vi "Tracking.vi"(4 "Offset Home 2 RCM":dbl[](array[numeric])=[0.0, 0.0, 0.0, 0.0], 5 "Trajectory Cluster":T3, 6 "PID Cluster":T6={"L1 to L4 PID Cluster"={"L1 PID Gains"={"Kp"=0.005, "Kd"=0.5, "Ki"=0.0005}, "L2 PID Gains"={"Kp"=0.01, "Kd"=1.0, "Ki"=0.005}, "L3 PID Gains"={"Kp"=0.05, "Kd"=1.0, "Ki"=0.0005}, "L4 PID Gains"={"Kp"=0.1, "Kd"=0.1, "Ki"=0.0005}}, "Stage PID Cluster"={"Stage Z PID"={"Kp"=0.0005, "Kd"=0.001, "Ki"=0.0}, "Stage Y PID"={"Kp"=0.0003, "Kd"=0.01, "Ki"=0.0}, "Stage X PID"={"Kp"=0.0003, "Kd"=0.01, "Ki"=0.0}}, "OCT Z PID Gains"={"Kp"=0.0003, "Kd"=0.0001, "Ki"=0.01}}, 7 "Eye Model Cluster":T2={"X Grid"=[], "Y Grid"=[], "Za_true Surf"=[], "Iris Center"=[], "Zp_true Surf"=[], "Pinv"=[[1.0, 0.0], [0.0, 1.0]], "za_true"=5.0, "za_work"=1.0, "zp_work"=-1.0, "zp_true"=-5.0}, 8 "error in":errorcluster, 9 "Resume Index":i32, 10 "Prev Posit Cluster":T5={"Prev L1 to L4 Posit"=[-0.5319, -0.035669172703475985, -2.0566170657346783, 0.9099264705882353], "Prev Stage Posit"=[6.002553885707208, 5.996566124542428, 5.995469940427586], "Prev OCT Z Posit"=-0.0}, 11 "FPGA VI Reference In":refnum<k20>) -> (0 "error out":errorcluster, 1 "Leave Index":i32, 2 "Last Posit Cluster":T4={"Last L1 to L4 Posit"=[0.0, 0.0, 0.0, 0.0], "Last Stage Posit"=[6.0, 6.0, 6.0], "Last OCT Z Posit"=0.0}, 3 "FPGA VI Reference Out":refnum<k20>)   [LabVIEW 2016]
uses:
  <vilib>/Analysis/Matrix/Datatypes/RealMatrix.ctl
  <vilib>/Platform/TimedLoop/XDataNode/timing_clust.ctl
  <vilib>/Platform/TimedLoop/XDataNode/nitl_modes.ctl
  <vilib>/Platform/TimedLoop/XDataNode/wakeup.ctl
  Global Variables.vi
  <vilib>/platform/TimedLoop/XDataNode/XDataNode.xnode
  <vilib>/Platform/TimedLoop/XDataNode/XDNodeRunTimeDep.lvlib
  Library/KevinLibraryAll/labview/KevLib01.lvlib
  <vilib>/Analysis/Matrix/NI_Matrix.lvlib
panel:
  out "PC z Displacement":dbl
  out "Speed Schedule":dbl
  out "In Servo Loop":bool
  out "joint limits":dbl[][](array[numeric])=[[-10.0, 35.0], [-35.0, 35.0], [0.1, 10.0], [-40.0, 40.0]]
  out "Vac Extremum":dbl[](array[numeric])
  out "z Dist Thld":dbl[](array[numeric])
  out "z Rot Axis":dbl
  out "Deform Array":dbl[](array[numeric])=[1.0, 1.0, 1.0, 0.0, 0.0, 0.0, 0.0, 0.0, 0.0]
  out "Speed Override":u16(ring)=3 items=["4x", "3x", "2x", "1x", "0.5x", "0.2x", "0.1x", "PAUSE"]
  out "Loading Finished":bool
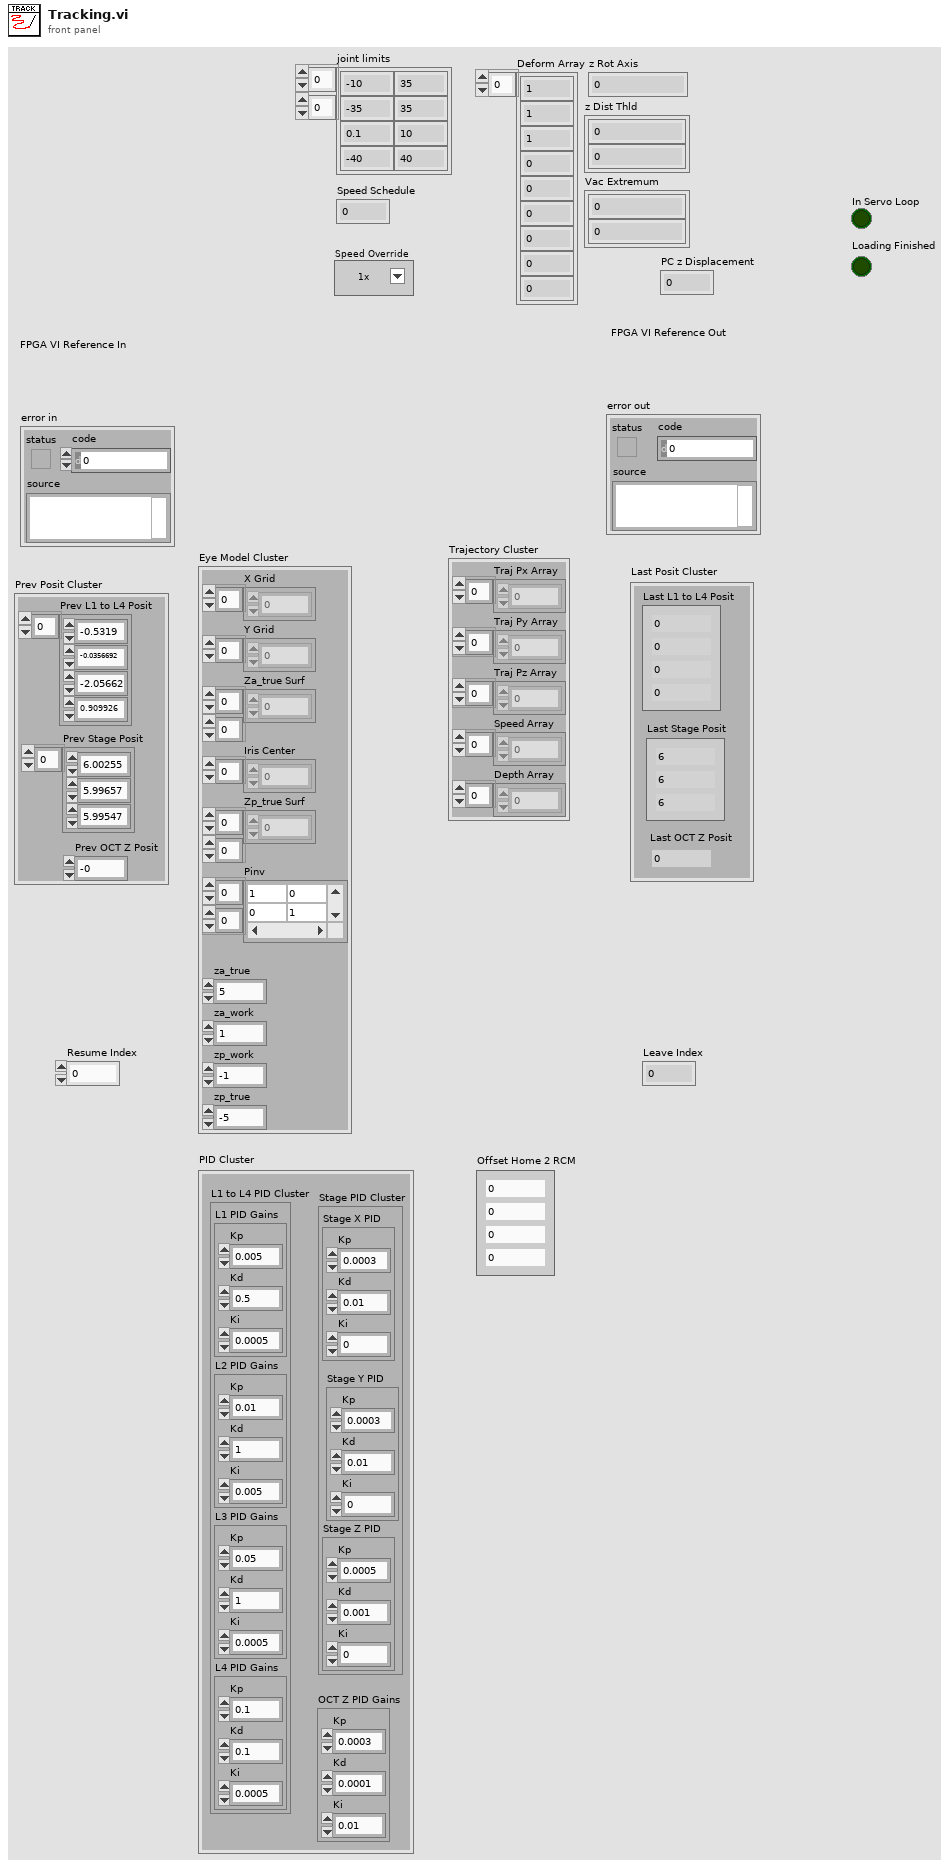
[diagram p1: front panel]
types:
  T1 = typedef "NI_Matrix.lvlib/RealMatrix.ctl" = dbl[][]
  T2 = cluster{"X Grid":dbl[], "Y Grid":dbl[], "Za_true Surf":dbl[][], "Iris Center":dbl[], "Zp_true Surf":dbl[][], "Pinv":T1, "za_true":dbl, "za_work":dbl, "zp_work":dbl, "zp_true":dbl}
  T3 = cluster{"Traj Px Array":dbl[], "Traj Py Array":dbl[], "Traj Pz Array":dbl[], "Speed Array":dbl[], "Depth Array":dbl[]}
  T4 = cluster{"Last L1 to L4 Posit":dbl[], "Last Stage Posit":dbl[], "Last OCT Z Posit":dbl}
  T5 = cluster{"Prev L1 to L4 Posit":dbl[], "Prev Stage Posit":dbl[], "Prev OCT Z Posit":dbl}
  T6 = cluster{"L1 to L4 PID Cluster":cluster{"L1 PID Gains":cluster{"Kp":dbl, "Kd":dbl, "Ki":dbl}, "L2 PID Gains":cluster{"Kp":dbl, "Kd":dbl, "Ki":dbl}, "L3 PID Gains":cluster{"Kp":dbl, "Kd":dbl, "Ki":dbl}, "L4 PID Gains":cluster{"Kp":dbl, "Kd":dbl, "Ki":dbl}}, "Stage PID Cluster":cluster{"Stage Z PID":cluster{"Kp":dbl, "Kd":dbl, "Ki":dbl}, "Stage Y PID":cluster{"Kp":dbl, "Kd":dbl, "Ki":dbl}, "Stage X PID":cluster{"Kp":dbl, "Kd":dbl, "Ki":dbl}}, "OCT Z PID Gains":cluster{"Kp":dbl, "Kd":dbl, "Ki":dbl}}
  T7 = typedef "XDNodeRunTimeDep.lvlib/timing_clust.ctl" = cluster{"Expected End [f-1]":u64, "Actual End [f-1]":u64, "Finished Late? [f-1]":bool, "Expected End [i-1]":u64, "Actual End [i-1]":u64, "Finished Late? [i-1]":bool, "Expected Start [i]":u64, "Actual Start [i]":u64, "Expected Start [f]":u64, "Actual Start [f]":u64, "Source Name":string, "Structure Name":string, "Period":i64, "Deadline":i64, "Offset":i64, "Start":i64, "Priority":i32, "Timeout":i32, "Mode":T8, "Wakeup Reason":T9, "Error":errorcluster, "Source Type":string, "Secondary Source Type":string, "Global End Time":u64, "Global Start Time":u64, "Frame Duration":u64, "Iteration Duration":u64, "Assigned CPU":i32, "I/O Scan Engine Mode":u32}
  T8 = typedef "XDNodeRunTimeDep.lvlib/nitl_modes.ctl" = enum32{"No Change", "Process missed periods, maintain original phase", "Discard missed periods, maintain original phase", "Process missed periods, ignore original phase", "Discard missed periods, ignore original phase"}
  T9 = typedef "XDNodeRunTimeDep.lvlib/wakeup.ctl" = enum32{"Normal", "Aborted", "Asynchronous wakeup", "Timing source error", "Timed loop error", "Timeout"}
  T10 = cluster{"Stop Vacuum":bool, "Vacuum Force":i8, "Max Limit [mmHg]":dbl, "Slide in":i8, "Irrigation?":bool}
  T11 = cluster{"L1 PID Gains":cluster{"Kp":dbl, "Kd":dbl, "Ki":dbl}, "L2 PID Gains":cluster{"Kp":dbl, "Kd":dbl, "Ki":dbl}, "L3 PID Gains":cluster{"Kp":dbl, "Kd":dbl, "Ki":dbl}, "L4 PID Gains":cluster{"Kp":dbl, "Kd":dbl, "Ki":dbl}}
  T12 = cluster{"Stage Z PID":cluster{"Kp":dbl, "Kd":dbl, "Ki":dbl}, "Stage Y PID":cluster{"Kp":dbl, "Kd":dbl, "Ki":dbl}, "Stage X PID":cluster{"Kp":dbl, "Kd":dbl, "Ki":dbl}}
  T13 = cluster{"Accurus button":bool[], "Accurus engaged?":bool, "Vacuum Force":i32, "Accurus Ch. A Vout":dbl, "Accurus Ch. B Vout":dbl, "Irrigation engaged?":bool}
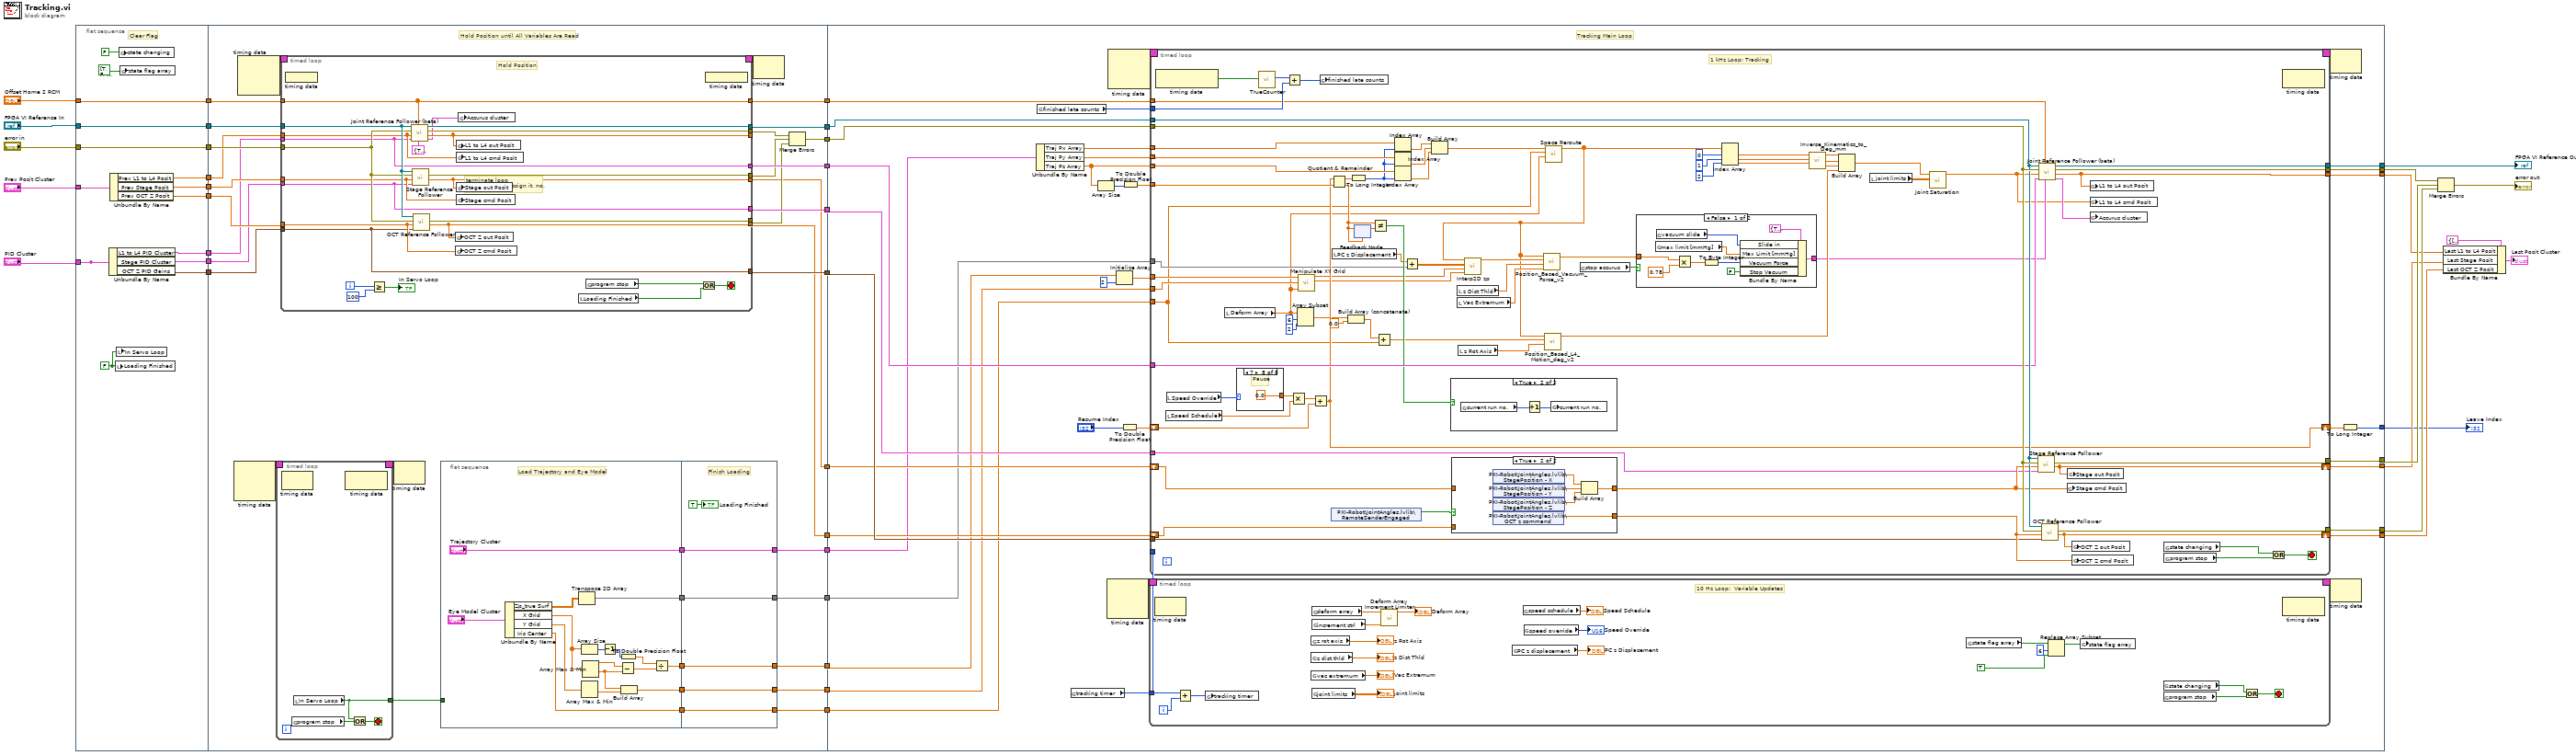
[diagram p0: block diagram]
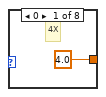
[diagram p2: hidden frame]
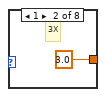
[diagram p3: hidden frame]
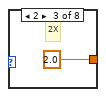
[diagram p4: hidden frame]
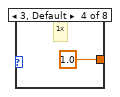
[diagram p5: hidden frame]
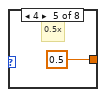
[diagram p6: hidden frame]
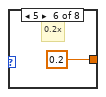
[diagram p7: hidden frame]
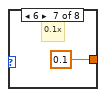
[diagram p8: hidden frame]
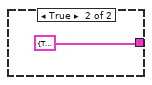
[diagram p9: hidden frame]
diagram:
  n1 = flat-sequence {
    tunnel: [w50] -> w38
    tunnel: "FPGA VI Reference In" -> [w50]
    tunnel: "error in" -> [w49]
    tunnel: [w49] -> w35
    tunnel: "Prev Posit Cluster" -> [w48]
    tunnel: [w47] -> _
    tunnel: "PID Cluster" -> [w47]
    tunnel: [w46] -> w32
    tunnel: [w45] -> w31
    tunnel: [w44] -> w30
    tunnel: [w43] -> w29
    tunnel: [w42] -> w28
    tunnel: "Offset Home 2 RCM" -> [w42]
    tunnel: [w41] -> w23
    tunnel: [w39] -> w6
    tunnel: w38 -> [w87]
    tunnel: w35 -> [w86]
    tunnel: w32 -> [w85]
    tunnel: w31 -> [w84]
    tunnel: w30 -> [w83]
    tunnel: w29 -> [w82]
    tunnel: w28 -> [w81]
    tunnel: [w80] -> w26
    tunnel: [w79] -> w25
    tunnel: [w78] -> w24
    tunnel: w23 -> [w77]
    tunnel: [w76] -> w22
    tunnel: [w75] -> w21
    tunnel: [w74] -> w20
    tunnel: [w73] -> w9
    tunnel: [w72] -> w8
    tunnel: [w71] -> w7
    tunnel: w6 -> [w70]
    tunnel: [w64] -> w5
    tunnel: [w63] -> w4
    tunnel: [w59] -> w2
    tunnel: [w58] -> w1
    tunnel: w26 -> [w179]
    tunnel: w25 -> [w145]
    tunnel: w24 -> [w178]
    tunnel: w22 -> [w176]
    tunnel: w21 -> [w175]
    tunnel: w20 -> [w174]
    tunnel: [w173] -> w16
    tunnel: [w172] -> w15
    tunnel: [w171] -> w14
    tunnel: [w170] -> w13
    tunnel: [w169] -> w12
    tunnel: [w168] -> w11
    tunnel: [w167] -> w10
    tunnel: w9 -> [w161]
    tunnel: w8 -> [w149]
    tunnel: w7 -> [w162]
    tunnel: w5 -> [w164]
    tunnel: w4 -> [w163]
    tunnel: [w157] -> w3
    tunnel: w2 -> [w150]
    tunnel: w1 -> [w151]
    frame #0 {
      w40 = FALSE ("Loading Finished")
      # "Clear Flag"
      n2 = Unbundle By Name(w47) -> ("L1 to L4 PID Cluster"=w43:T11, "Stage PID Cluster"=w41:T12, "OCT Z PID Gains"=w46:cluster{"Kp":dbl, "Kd":dbl, "Ki":dbl})
      n3 = Unbundle By Name(w48) -> ("Prev L1 to L4 Posit"=w39:dbl[], "Prev Stage Posit"=w45:dbl[], "Prev OCT Z Posit"=w44:dbl)
      n4 = local write "Loading Finished"(w40) -> ()
      n5 = local write "In Servo Loop"(w40) -> ()
      n6 = global write "Global Variables.vi" "state changing"(FALSE ("state changing")) -> ()
      n7 = global write "Global Variables.vi" "state flag array"(bool[] [TRUE, FALSE, FALSE, FALSE, FALSE, FALSE, FALSE, FALSE, FALSE] ("state flag array")) -> ()
    }
    frame #1 {
      # "terminate loop\nwhen it. no. > assign it. no."
      # "Hold Position until All Variables Are Read"
      n8 = node-c288() -> (w62:T7)  [unwired: 3 in]
      n9 = node-c288() -> (w69:T7)  [unwired: 3 in]
      n10 = timed-loop {
        timing: w62 -> [_]
        timing-out: [_] -> w61
        tunnel: [w110] -> w60
        stop <- w112 stop-if-true
        n11 = node-c288() -> ()  [unwired: 1 in, 1 out]
        n12 = global read "Global Variables.vi" "program stop"() -> (w111:bool)
        n13 = local read "In Servo Loop"() -> (w110:bool)
        n14 = node-c288() -> ()  [unwired: 1 in, 1 out]
        n15 = Or(x=w110, y=w111) -> (x .or. y?=w112:bool)
      }
      n16 = timed-loop {
        timing: w69 -> [_]
        timing-out: [_] -> w68
        tunnel: [w137] -> _
        tunnel: [w136] -> w64
        tunnel: [w135] -> w63
        tunnel: [w134] -> w80
        tunnel: [w133] -> w67
        tunnel: [w132] -> w66
        tunnel: [w131] -> w65
        tunnel: w87 -> [w130]
        tunnel: w86 -> [w129]
        tunnel: w85 -> [w124]
        tunnel: w70 -> [w127]
        tunnel: w84 -> [w128]
        tunnel: w83 -> [w126]
        tunnel: w82 -> [w122]
        tunnel: w81 -> [w125]
        tunnel: [w125] -> w79
        tunnel: w77 -> [w123]
        tunnel: [w124] -> w74
        tunnel: [w123] -> w75
        tunnel: [w122] -> w76
        i -> [w121]
        stop <- w140 stop-if-true
        # "Hold Position"
        n17 = node-c288 ("Output Node")() -> ()  [unwired: 1 in]
        n18 = Greater Or Equal?(x=w121, y=100) -> (x >= y?=→"In Servo Loop":bool)
        n19 = call "Joint Reference Follower (beta).vi"("Accurus Ctrl Cluster"=T10 {"Stop Vacuum"=TRUE, "Vacuum Force"=0, "Max Limit [mmHg]"=600.0, "Slide in"=0, "Irrigation?"=TRUE}, "Offset Home2RCM [deg/mm]"=w125, "PID Ctrl Cluster"=w122, "Ref Array [deg/mm]"=w127, "error in"=w129, "FPGA VI Reference In"=w130) -> ("Accurus Output Cluster"=w117:T13, "Output Posit Array [deg/mm]"=w137:dbl[], "error out"=w133:errorcluster, "FPGA VI Reference Out"=w134:refnum<k20>)  [unwired: 2 in]
        n20 = call "Stage Reference Follower.vi"("Stage PID Cluster"=w123, "Stage cmd Posit [mm]"=w128, "error in"=w129, "FPGA VI Reference In"=w130) -> ("Stage out Posit [mm]"=w136:dbl[], "error out"=w132:errorcluster)  [unwired: 5 in, 1 out]
        n21 = call "OCT Reference Follower.vi"("OCT Z PID Gains"=w124, "OCT  Z cmd Posit [mm]"=w126, "error in"=w129, "FPGA VI Reference In"=w130) -> ("OCT  Z out Posit [mm]"=w135:dbl, "error out"=w131:errorcluster)  [unwired: 5 in, 1 out]
        n22 = global write "Global Variables.vi" "OCT Z out Posit"(w135) -> ()
        n23 = global write "Global Variables.vi" "OCT Z cmd Posit"(w126) -> ()
        n24 = global write "Global Variables.vi" "L1 to L4 out Posit"(w137) -> ()
        n25 = global write "Global Variables.vi" "L1 to L4 cmd Posit"(w127) -> ()
        n26 = global write "Global Variables.vi" "Stage out Posit"(w136) -> ()
        n27 = global write "Global Variables.vi" "Stage cmd Posit"(w128) -> ()
        n28 = global write "Global Variables.vi" "Accurus cluster"(w117) -> ()
        n29 = local read "Loading Finished"() -> (w139:bool)
        n30 = global read "Global Variables.vi" "program stop"() -> (w138:bool)
        n31 = Or(x=w138, y=w139) -> (x .or. y?=w140:bool)
        n32 = node-c288() -> ()  [unwired: 1 out]
      }
      n33 = node-c288(w61) -> ()  [unwired: 1 out]
      n34 = flat-sequence {
        tunnel: [w90] -> w57
        tunnel: [w103] -> w56
        tunnel: [w102] -> w55
        tunnel: [w89] -> w54
        tunnel: ["Trajectory Cluster"] -> w53
        tunnel: w60 -> [_]
        tunnel: [w107] -> w71
        tunnel: [w108] -> w72
        tunnel: [w109] -> w73
        tunnel: w57 -> [w109]
        tunnel: w56 -> [w108]
        tunnel: w55 -> [w107]
        tunnel: w54 -> [w105]
        tunnel: [w105] -> w59
        tunnel: [w104] -> w58
        tunnel: w53 -> [w104]
        frame #0 {
          # "Load Trajectory and Eye Model"
          n35 = Unbundle By Name("Eye Model Cluster") -> ("Zp_true Surf"=w91:dbl[][], "X Grid"=w92:dbl[], "Y Grid"=w101:dbl[], "Iris Center"=w89:dbl[])
          n36 = Transpose 2D Array(2D array=w91) -> (transposed array=w90:dbl[][])
          n37 = Array Size(array=w92) -> (size(s)=w100:i32)
          n38 = Array Max & Min(array=w101) -> (min value=w97:dbl)  [unwired: 3 out]
          n39 = Array Max & Min(array=w92) -> (max value=w98:dbl, min value=w99:dbl)  [unwired: 2 out]
          n40 = Decrement(x=w100) -> (x-1=w95:i32)
          n41 = Subtract(x=w98, y=w99) -> (x-y=w94:dbl)
          n42 = To Double Precision Float(number=w95) -> (double precision float=w96:dbl)
          n43 = Build Array(w99, w97) -> (w102:dbl[])
          n44 = Divide(x=w96, y=w94) -> (x/y=w103:dbl)
        }
        frame #1 {
          # "Finish Loading"
          "Loading Finished" <- TRUE ("Loading Finished")
        }
      }
      n45 = node-c288(w68) -> ()  [unwired: 1 out]
      n46 = Merge Errors(w67, w66, w65) -> (w78:errorcluster)
    }
    frame #2 {
      # "Tracking Main Loop"
      n47 = Unbundle By Name(w151) -> ("Traj Px Array"=w160:dbl[], "Traj Py Array"=w159:dbl[], "Traj Pz Array"=w154:dbl[])
      n48 = global read "Global Variables.vi" "finished late counts"() -> (w177:u16)
      n49 = global read "Global Variables.vi" "tracking timer"() -> (w146:i32)
      n50 = Array Size(array=w154) -> (size(s)=w153:i32)
      n51 = node-c288() -> (w166:T7)  [unwired: 3 in]
      n52 = node-c288() -> (w181:T7)  [unwired: 3 in]
      n53 = Initialize Array(w149, 2 ("dimension size")) -> (w147:dbl[])
      n54 = To Double Precision Float(number="Resume Index") -> (double precision float=w156:dbl)
      n55 = To Double Precision Float(number=w153) -> (double precision float=w152:dbl)
      n56 = timed-loop {
        timing: w166 -> [_]
        timing-out: [_] -> w165
        tunnel: w146 -> [w182]
        i -> [w183]
        stop <- w201 stop-if-true
        # "10 Hz Loop:  Variable Updates"
        n57 = node-c288() -> ()  [unwired: 1 in, 1 out]
        n58 = Add(x=w182, y=w183) -> (x+y=w184:i32)
        n59 = global write "Global Variables.vi" "tracking timer"(w184) -> ()
        n60 = global read "Global Variables.vi" "z rot axis"() -> (→"z Rot Axis":dbl)
        n61 = global read "Global Variables.vi" "z dist thld"() -> (→"z Dist Thld":dbl[])
        n62 = global read "Global Variables.vi" "vac extremum"() -> (→"Vac Extremum":dbl[])
        n63 = global read "Global Variables.vi" "deform array"() -> (w191:dbl[])
        n64 = global read "Global Variables.vi" "increment ctrl"() -> (w190:dbl[])
        n65 = global read "Global Variables.vi" "joint limits"() -> (→"joint limits":dbl[][])
        n66 = call "Deform Array Increment Limiter.vi"("Increment Array"=w190, "Defrom Ref"=w191) -> ("Deform Output"=→"Deform Array":dbl[])  [unwired: 9 in]
        n67 = global read "Global Variables.vi" "PC z displacement"() -> (→"PC z Displacement":dbl)
        n68 = global read "Global Variables.vi" "speed schedule"() -> (→"Speed Schedule":dbl)
        n69 = global read "Global Variables.vi" "speed override"() -> (→"Speed Override":u16)
        n70 = global read "Global Variables.vi" "state flag array"() -> (w187:bool[])
        n71 = Replace Array Subset(array=w187, new element=TRUE ("new element/subarray"), index=6) -> (w188:bool[])
        n72 = global write "Global Variables.vi" "state flag array"(w188) -> ()
        n73 = global read "Global Variables.vi" "state changing"() -> (w200:bool)
        n74 = global read "Global Variables.vi" "program stop"() -> (w199:bool)
        n75 = Or(x=w200, y=w199) -> (x .or. y?=w201:bool)
        n76 = node-c288() -> ()  [unwired: 1 in, 1 out]
      }
      n77 = timed-loop {
        timing: w181 -> [_]
        timing-out: [_] -> w180
        tunnel: w160 -> [w286]
        tunnel: w159 -> [w285]
        tunnel: w154 -> [w253]
        tunnel: w179 -> [w279]
        tunnel: w145 -> [w264]
        tunnel: w178 -> [w280]
        tunnel: [w281] -> w173
        tunnel: w176 -> [w262]
        tunnel: w177 -> [w275]
        tunnel: w175 -> [w257]
        tunnel: w174 -> [w261]
        shift-right: [w273] -> w168
        shift-left: w164 -> [w271]
        shift-right: [w272] -> w167
        shift-left: w163 -> [w270]
        tunnel: [w268] -> w171
        tunnel: [w267] -> w170
        tunnel: [w266] -> w172
        tunnel: [w263] -> w169
        shift-right: [w229] -> w158
        shift-left: w156 -> [w234]
        tunnel: w161 -> [w219]
        tunnel: w147 -> [w225]
        tunnel: w162 -> [w224]
        tunnel: w152 -> [w232]
        tunnel: w150 -> [w212]
        tunnel: w146 -> [_]
        stop <- w282 stop-if-true
        # "1 kHz Loop: Tracking"
        n78 = node-c288() -> (w278:bool)  [unwired: 1 in]
        n79 = local read "Speed Schedule"() -> (w237:dbl)
        n80 = local read "Speed Override"() -> (w236:u16)
        n81 = local read "Deform Array"() -> (w218:dbl[])
        n82 = case shown="7" w236 {
          tunnel: [4.0 ("y") 3.0 ("y") 2.0 ("y") 1.0 ("y") 0.5 ("y") 0.2 ("y") 0.1 ("y") 0.0 ("y")] -> w235
          frame 0 {
            # "4X"
          }
          frame 1 {
            # "3X"
          }
          frame 2 {
            # "2X"
          }
          frame 3, Default {
            # "1x"
          }
          frame 4 {
            # "0.5x"
          }
          frame 5 {
            # "0.2x"
          }
          frame 6 {
            # "0.1x"
          }
          frame 7 {
            # "Pause"
          }
        }
        n83 = call "TrueCounter.vi"("True?"=w278) -> ("True Count"=w276:u16)  [unwired: 10 in]
        n84 = Add(x=w276, y=w275) -> (x+y=w277:u16)
        n85 = Multiply(x=w235, y=w237) -> (x*y=w238:dbl)
        n86 = Array Subset(array=w218, index=6, length=2) -> (w215:dbl[])
        n87 = call "Manipulate XY Grid.vi"("Deform Array"=w218, "XY Grid min In"=w224, "XY Quant. Fact. In"=w225) -> ("XY Grid min Out"=w221:dbl[], "XY Quant. Fact. Out"=w222:dbl[])  [unwired: 7 in]
        n88 = Add(x=w238, y=w234) -> (x+y=w229:dbl)
        n89 = global write "Global Variables.vi" "finished late counts"(w277) -> ()
        n90 = Quotient & Remainder(x=w229, y=w232) -> (x-y*floor(x/y)=w231:dbl, floor(x/y)=w226:dbl)
        n91 = shared-variable "PXI-Robot\\JointAngles.lvlib\\RemoteSenderEngaged"() -> (w274:bool)  [unwired: 1 in, 1 out]
        n92 = local read "PC z Displacement"() -> (w220:dbl)
        n93 = Build Array (concatenate)(w215, 0.0) -> (w214:dbl[])
        n94 = To Long Integer(number=w231) -> (32bit integer=w230:i32)
        n95 = feedback-in #1(w226) -> ()
        n96 = feedback #1(w226) -> (w228:dbl)
        n97 = Not Equal?(x=w226, y=w228) -> (x != y?=w227:bool)
        n98 = Add(x=w214, y=w212) -> (x+y=w208:dbl[])
        n99 = Index Array(array=w286, index=w230) -> (element=w242:dbl)
        n100 = Index Array(array=w285, index=w230) -> (element=w241:dbl)
        n101 = Index Array(array=w253, index=w230) -> (element=w240:dbl)
        n102 = Add(x=w220, y=w219) -> (x+y=w223:dbl[][])
        n103 = Build Array(w242, w241, w240) -> (w209:dbl[])
        n104 = case shown="True" w227 {
          frame False {
          }
          frame True {
            n105 = global read "Global Variables.vi" "current run no."() -> (w306:u8)
            n106 = Increment(x=w306) -> (x+1=w305:u8)
            n107 = global write "Global Variables.vi" "current run no."(w305) -> ()
          }
        }
        n108 = case shown="True" w274 {
          tunnel: [w308 w310] -> w269
          tunnel: [w307 w309] -> w265
          tunnel: w271 -> [w308 _]
          tunnel: w270 -> [w307 _]
          frame False {
            # "Hold Position if not Engaged"
          }
          frame True {
            n109 = shared-variable "PXI-Robot\\JointAngles.lvlib\\StagePosition - X"() -> (w313:dbl)  [unwired: 1 in, 1 out]
            n110 = shared-variable "PXI-Robot\\JointAngles.lvlib\\StagePosition - Y"() -> (w312:dbl)  [unwired: 1 in, 1 out]
            n111 = shared-variable "PXI-Robot\\JointAngles.lvlib\\StagePosition - Z"() -> (w311:dbl)  [unwired: 1 in, 1 out]
            n112 = shared-variable "PXI-Robot\\JointAngles.lvlib\\OCT z command"() -> (w309:dbl)  [unwired: 1 in, 1 out]
            n113 = Build Array(w313, w312, w311) -> (w310:dbl[])
          }
        }
        n114 = local read "z Dist Thld"() -> (w256:dbl[])
        n115 = local read "Vac Extremum"() -> (w255:dbl[])
        n116 = local read "z Rot Axis"() -> (w250:dbl)
        n117 = call "Space Reroute.vi"("Deform Array"=w218, "Pivot Pt"=w212, "Nominal Traj Pt"=w209) -> ("Reroute Traj Pt"=w207:dbl[])  [unwired: 8 in]
        n118 = call "Interp2D zp.vi"("XY Grid min"=w221, "XY Quantization Factor"=w222, "Zp array"=w223, "Tip Position"=w207) -> ("zp"=w233:dbl)  [unwired: 7 in]
        n119 = call "Position_Based_Vacuum_Force_v2.vi"("vac_bnd"=w255, "z_thld"=w256, "current zp"=w233, "tip position"=w207) -> ("vacf (%)"=w254:dbl)  [unwired: 7 in]
        n120 = call "Position_Based_L4_Motion_deg_v2.vi"("Assign z"=w250, "Iris Center"=w208, "Tip Position"=w207) -> ("L4 Motion [deg]"=w249:dbl)  [unwired: 8 in]
        n121 = global read "Global Variables.vi" "stop accurus"() -> (w239:bool)
        n122 = case shown="False" w239 {
          tunnel: [w297 T10 {"Stop Vacuum"=TRUE, "Vacuum Force"=0, "Max Limit [mmHg]"=600.0, "Slide in"=0, "Irrigation?"=TRUE} ("Accurus Ctrl Cluster")] -> w211
          tunnel: w254 -> [w296 _]
          frame False {
            n123 = global read "Global Variables.vi" "max limit [mmHg]"() -> (w301:dbl)
            n124 = global read "Global Variables.vi" "vacuum slide"() -> (w302:i8)
            n125 = Multiply(x=w296, y=0.78 ("x")) -> (x*y=w299:dbl)
            n126 = To Byte Integer(number=w299) -> (8bit integer=w298:i8)
            n127 = Bundle By Name(cluster=T10 {"Stop Vacuum"=TRUE, "Vacuum Force"=0, "Max Limit [mmHg]"=600.0, "Slide in"=0, "Irrigation?"=TRUE} ("Accurus Ctrl Cluster"), "Slide in"=w302, "Max Limit [mmHg]"=w301, "Vacuum Force"=w298, "Stop Vacuum"=FALSE ("Stop Accurus")) -> (w297:T10)
          }
          frame True {
          }
        }
        n128 = Index Array(array=w207, index #1=0 ("index"), index #2=1 ("index"), index #3=2 ("index")) -> (element #1=w245:dbl, element #2=w244:dbl, element #3=w243:dbl)
        n129 = call "Inverse_Kinematics_to_Deg_mm.vi"("pz"=w243, "py"=w244, "px"=w245) -> ("L3 [mm]"=w259:dbl, "L2 [deg]"=w260:dbl, "L1 [deg]"=w284:dbl)
        n130 = Build Array(w284, w260, w259, w249) -> (w252:dbl[])
        n131 = local read "joint limits"() -> (w251:dbl[][])
        n132 = call "Joint Saturation.vi"("Joint Bounds [Deg/mm]"=w251, "Ref Array [Deg/mm]"=w252) -> ("Sat Ref Array [Deg/mm]"=w206:dbl[])  [unwired: 9 in]
        n133 = call "Stage Reference Follower.vi"("Stage PID Cluster"=w257, "Stage cmd Posit [mm]"=w269, "error in"=w280, "FPGA VI Reference In"=w279) -> ("Stage out Posit [mm]"=w273:dbl[], "error out"=w268:errorcluster)  [unwired: 5 in, 1 out]
        n134 = call "Joint Reference Follower (beta).vi"("Accurus Ctrl Cluster"=w211, "Offset Home2RCM [deg/mm]"=w264, "PID Ctrl Cluster"=w262, "Ref Array [deg/mm]"=w206, "error in"=w280, "FPGA VI Reference In"=w279) -> ("Accurus Output Cluster"=w210:T13, "Output Posit Array [deg/mm]"=w263:dbl[], "error out"=w266:errorcluster, "FPGA VI Reference Out"=w281:refnum<k20>)  [unwired: 2 in]
        n135 = call "OCT Reference Follower.vi"("OCT Z PID Gains"=w261, "OCT  Z cmd Posit [mm]"=w265, "error in"=w280, "FPGA VI Reference In"=w279) -> ("OCT  Z out Posit [mm]"=w272:dbl, "error out"=w267:errorcluster)  [unwired: 5 in, 1 out]
        n136 = global write "Global Variables.vi" "Stage cmd Posit"(w269) -> ()
        n137 = global write "Global Variables.vi" "Stage out Posit"(w273) -> ()
        n138 = global write "Global Variables.vi" "OCT Z out Posit"(w272) -> ()
        n139 = global write "Global Variables.vi" "OCT Z cmd Posit"(w265) -> ()
        n140 = global write "Global Variables.vi" "L1 to L4 out Posit"(w263) -> ()
        n141 = global write "Global Variables.vi" "L1 to L4 cmd Posit"(w206) -> ()
        n142 = global write "Global Variables.vi" "Accurus cluster"(w210) -> ()
        n143 = global read "Global Variables.vi" "state changing"() -> (w258:bool)
        n144 = global read "Global Variables.vi" "program stop"() -> (w283:bool)
        n145 = Or(x=w258, y=w283) -> (x .or. y?=w282:bool)
        n146 = node-c288() -> ()  [unwired: 1 in, 1 out]
      }
      n147 = node-c288(w180) -> ()  [unwired: 1 out]
      n148 = node-c288(w165) -> ()  [unwired: 1 out]
      n149 = To Long Integer(number=w158) -> (32bit integer=w157:i32)
    }
  }
  n150 = Merge Errors(w15, w14, w13) -> (→"error out":errorcluster)
  n151 = Bundle By Name(cluster=T4 {"Last L1 to L4 Posit"=[0.0, 0.0, 0.0, 0.0], "Last Stage Posit"=[6.0, 6.0, 6.0], "Last OCT Z Posit"=0.0} ("Last Posit Cluster 2"), "Last L1 to L4 Posit"=w12, "Last Stage Posit"=w11, "Last OCT Z Posit"=w10) -> (→"Last Posit Cluster":T4)
  "FPGA VI Reference Out" <- w16
  "Leave Index" <- w3
